vi "equals.vi"(8 "error in (no error)":errorcluster, 10 "Category to Match":refnum<class "Category.lvclass">, 11 "Category in":refnum<class "Category.lvclass">) -> (0 "error out":errorcluster, 2 "Equals?":bool, 3 "Category out":refnum<class "Category.lvclass">)   [LabVIEW 2018, in "Category.lvclass"]
uses:
  Category.lvclass
  Category.lvclass/Category.ctl
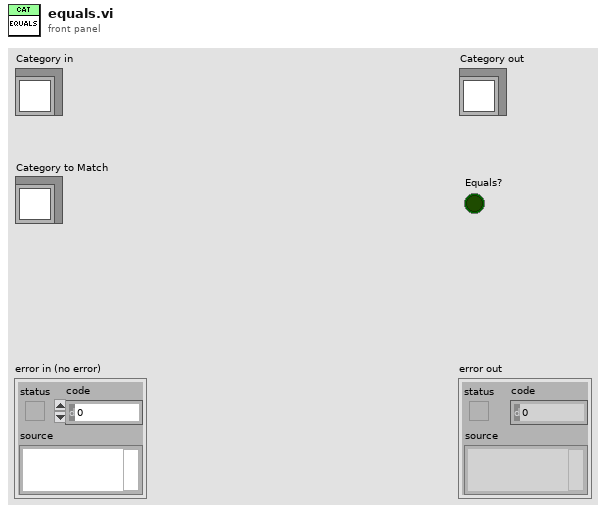
[diagram p1: front panel]
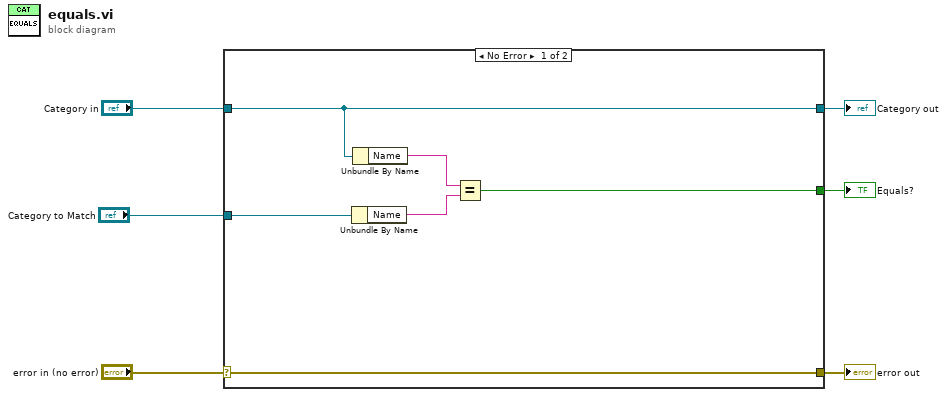
[diagram p0: block diagram]
diagram:
  n1 = case shown="No Error" "error in (no error)" {
    selector: "error in (no error)" -> [w12 w14]
    tunnel: [w12 w14] -> w5
    tunnel: [w11 w13] -> w3
    tunnel: "Category in" -> [w11 w13]
    tunnel: "Category to Match" -> [w10 _]
    tunnel: [w7 _] -> w1
    frame No Error {
      n2 = Unbundle By Name(w10) -> ("Name"=w8:string)
      n3 = Unbundle By Name(w11) -> ("Name"=w9:string)
      n4 = Equal?(x=w9, y=w8) -> (x = y?=w7:bool)
    }
    frame Error {
    }
  }
  "error out" <- w5
  "Category out" <- w3
  "Equals?" <- w1
